vi "Replace Image - Coloring.vi"(8 "error in":errorcluster, 10 "File with Button":path=path "C:/Users/daniel.coons/OneDrive - Technology Service Corporation/Desktop/button editor/button ui.vi", 11 "Material-Scheme":refnum<class "Material-Scheme.lvclass">) -> (0 "error out":errorcluster, 2 "File with Button (dup)":path=path "C:/Users/daniel.coons/OneDrive - Technology Service Corporation/Desktop/button editor/button ui.vi")   [LabVIEW 2021]
doc: "This example VI was obtained from this post: \n\nhttps://forums.ni.com/t5/LabVIEW-APIs-Discussions/Set-TRUE-FALSE-Image-of-a-boolean-control-automatically-using/m-p/3419083/highlight/true#M868\n\n<b>Code Developed By:</b>\nTechnology Service Corporation\n1983 S Liberty Drive\nBloomington, IN 47403\nPhone: 812 558-7100\ncustomtest.tsc.com\n\nDeveloper:\nDaniel Coons"
uses:
  Material-Scheme.lvclass
panel:
  # "MNGI resources are 6 images\non buttons (pressed, hover, etc)"
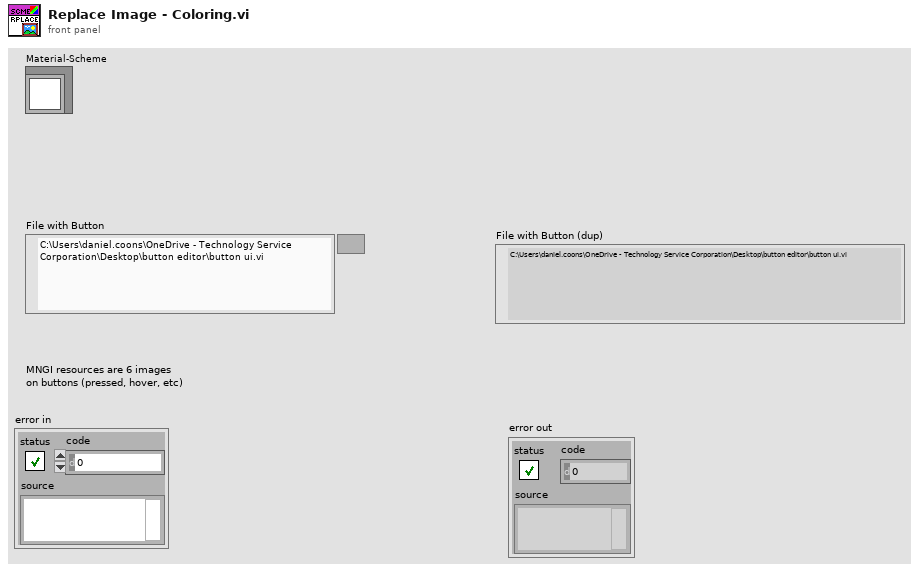
[diagram p1: front panel]
types:
  T1 = cluster{"type":u32, "id":i32, "name":string, "binary data":string}[]
  T2 = enum16{"open", "replace", "create", "open or create", "replace or create", "replace or create with confirmation"}
  T3 = cluster{"type":u32, "id":i32, "name":string, "binary data":string}
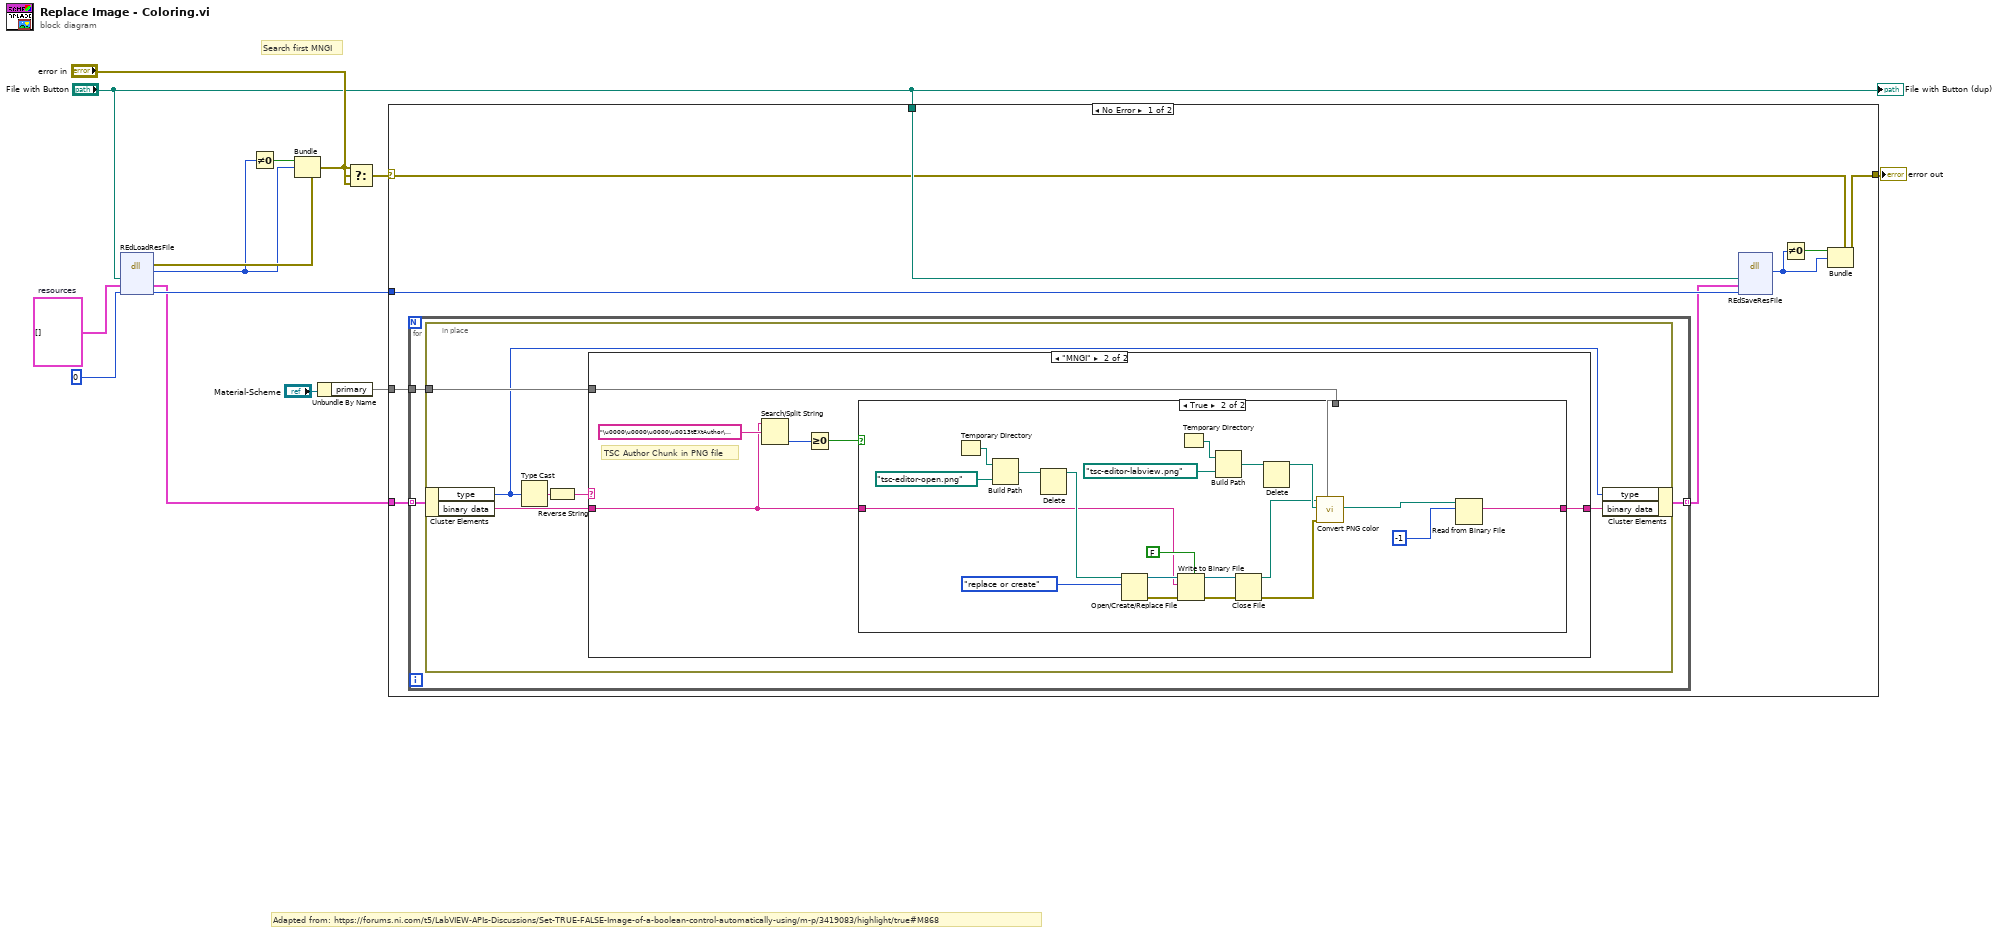
[diagram p0: block diagram]
diagram:
  w13 = T1 []  # resources
  # "Adapted from: https://forums.ni.com/t5/LabVIEW-APIs-Discussions/Set-TRUE-FALSE-Image-of-a-boolean-control-automatically-using/m-p/3419083/highlight/true#M868"
  # "Search first MNGI"
  n1 = dll-call lib="LabVIEW" fn="REdLoadResFile"("path"="File with Button", "resources"=w13, "type"=0) -> (error out=w11:errorcluster, "return type"=w9:i32, "resources"=w2:T1, "type"=w8:i32)  [unwired: 3 in, 2 out]
  n2 = Not Equal To 0?(x=w9) -> (x != 0?=w10:bool)
  n3 = Bundle(cluster=w11, "status"=w10, "code"=w9) -> (w6:errorcluster)  [unwired: 1 out]
  n4 = Unbundle By Name("Material-Scheme") -> ("primary"=w1)
  n5 = Select(t=w6, s=w6, f="error in") -> (s? t:f=w5:errorcluster)
  n6 = case shown="No Error" w5 {
    selector: w5 -> [w21 w62]
    tunnel: [w20 w62] -> w14
    tunnel: "File with Button" -> [w23 _]
    tunnel: w8 -> [w22 _]
    tunnel: w2 -> [w17 _]
    tunnel: w1 -> [w16 _]
    frame No Error {
      n7 = for {
        tunnel: w17 -> [w25] mode=indexing
        tunnel: w16 -> [w26]
        tunnel: [w24] -> w15 mode=indexing
        n8 = in-place {
          in-place-border: w26 -> [w30]
          n9 = in-place-cluster #1(w25) -> ("type"=w27:u32, "binary data"=w29:string)
          n10 = Type Cast(x=w27) -> (*(type *) &x=w32:string)  [unwired: 1 out]
          n11 = Reverse String(1:w32) -> (0:w31:string)
          n12 = case shown="\"MNGI\"" w31 {
            tunnel: w29 -> [w33 w35]
            tunnel: w30 -> [_ w36]
            tunnel: [w33 w34] -> w28
            frame Default {
            }
            frame "MNGI" {
              # "TSC Author Chunk in PNG file"
              n13 = Search/Split String(string=w35, search string/char (-)="\u0000\u0000\u0000\u0013tEXtAuthor\u0000tscicondecal^Ø" ("string")) -> (offset of match=w39:i32)  [unwired: 1 in, 2 out]
              n14 = Greater Or Equal To 0?(x=w39) -> (x >= 0?=w37:bool)
              n15 = case shown="True" w37 {
                tunnel: w35 -> [w40 w51]
                tunnel: w36 -> [_ w42]
                tunnel: [w40 w43] -> w34
                frame False {
                }
                frame True {
                  n16 = Temporary Directory() -> (w61:path)
                  n17 = Build Path(base path=w61, name or relative path=path "tsc-editor-open.png") -> (appended path=w59:path)
                  n18 = Delete(path (use dialog)=w59) -> (deleted path=w53:path)  [unwired: 4 in, 2 out]
                  n19 = Open/Create/Replace File(file path (use dialog)=w53, operation (0:open)=T2."replace or create") -> (refnum out=w56:refnum<file>, error out=w57:errorcluster)  [unwired: 4 in, 1 out]
                  n20 = Write to Binary File(file (use dialog)=w56, data=w51, error in=w57, 5:FALSE ("prepend array or string size? (T)")) -> (refnum out=w54:refnum<file>, error out=w55:errorcluster)  [unwired: 2 in, 1 out]
                  n21 = Temporary Directory() -> (w47:path)
                  n22 = Build Path(base path=w47, name or relative path=path "tsc-editor-labview.png") -> (appended path=w49:path)
                  n23 = Close File(refnum=w54, error in=w55) -> (path=w41:path, error out=w50:errorcluster)
                  n24 = Delete(path (use dialog)=w49) -> (deleted path=w46:path)  [unwired: 4 in, 2 out]
                  n25 = call "Convert PNG color.vi"("New Color"=w42, "error in"=w50, "new file"=w46, "orig file"=w41) -> ("new file out"=w45:path)  [unwired: 5 in, 2 out]
                  n26 = Read from Binary File(10:-1 ("count (1)"), 11:w45) -> (2:w43:string)  [unwired: 1 in, 6 out]
                }
              }
            }
          }
          n27 = in-place-cluster #1("type"=w27, "binary data"=w28) -> (w24:T3)
        }
      }
      n28 = dll-call lib="LabVIEW" fn="REdSaveResFile"("path"=w23, "resources"=w15, "type"=w22) -> ("return type"=w18:i32)  [unwired: 6 in, 2 out]
      n29 = Not Equal To 0?(x=w18) -> (x != 0?=w19:bool)
      n30 = Bundle(cluster=w21, "status"=w19, "code"=w18) -> (w20:errorcluster)  [unwired: 1 out]
    }
    frame Error {
    }
  }
  "error out" <- w14
  "File with Button (dup)" <- "File with Button"
